vi "First step for time diagram.vi"(5 "Время в милисикундах":i32, 8 "right vertical (0 or 1)":i32[](array[numeric]), 9 "right vertical (time)":i32[](array[numeric]), 10 "right gorizontal (0 or 1)":i32[](array[numeric]), 11 "right gorizontal (time)":i32[](array[numeric])) -> (0 "left vertical (0 or 1)":i32[](array[numeric]), 1 "left vertical (time)":i32[](array[numeric]), 2 "left gorizontal (0 or 1)":i32[](array[numeric]), 3 "left gorizontal (time)":i32[](array[numeric]))   [LabVIEW 2012]
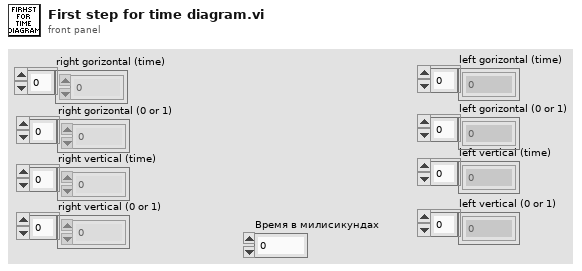
[diagram p1: front panel]
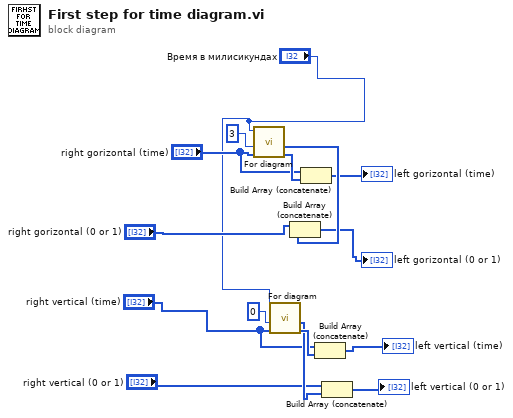
[diagram p0: block diagram]
diagram:
  n1 = call "For diagram.vi"("Предыдущий массив"="right gorizontal (time)", "Номер импульса"=3, "Время в милисикундах"="Время в милисикундах") -> ("Кол-во точек (время в милисек)"=w14:i32[], "Номер импульса (0 или 1)"=w13:i32[])  [unwired: 7 in]
  n2 = call "For diagram.vi"("Предыдущий массив"="right vertical (time)", "Номер импульса"=0, "Время в милисикундах"="Время в милисикундах") -> ("Кол-во точек (время в милисек)"=w11:i32[], "Номер импульса (0 или 1)"=w10:i32[])  [unwired: 7 in]
  n3 = Build Array (concatenate)("right gorizontal (0 or 1)", w13) -> (→"left gorizontal (0 or 1)":i32[])
  n4 = Build Array (concatenate)("right gorizontal (time)", w14) -> (→"left gorizontal (time)":i32[])
  n5 = Build Array (concatenate)("right vertical (time)", w11) -> (→"left vertical (time)":i32[])
  n6 = Build Array (concatenate)("right vertical (0 or 1)", w10) -> (→"left vertical (0 or 1)":i32[])
